vi "Cangrabber.vi"(8 "rt fifo":refnum<k33>) -> ()   [LabVIEW 2014]
uses:
  TeleopCmd.ctl
  CmdFlag.ctl
  <vilib>/Rock Robotics/Network Tables/SD Read Number.vi
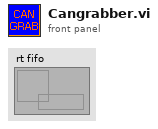
[diagram p1: front panel]
types:
  T1 = typedef "WPI_MotorControlDeviceRef.ctl" = cluster{"DeviceStatus":errorcluster, "Type":T2, "PWM":cluster{"Controller":T3, "PWM Channel":T4, "DeadBand":T5}, "CAN":cluster{"Device Number":u8, "Control Mode":T6, "Semaphore":T7, "Max Vout":dbl, "TalonSRX Control Mode":T8}, "Invert":bool, "TransformRef":T9, "InvTransformRef":T9}
  T2 = typedef "WPI_MotorControlType.ctl" = enum16{"PWM", "CAN", "CANTalonSRX"}
  T3 = typedef "FPGA_TypedefDigitalModule.ctl" = enum16{"Controller 1"}
  T4 = typedef "FPGA_DIOPWMChannel.ctl" = enum8{"PWM 0", "PWM 1", "PWM 2", "PWM 3", "PWM 4", "PWM 5", "PWM 6", "PWM 7", "PWM 8", "PWM 9", "PWM MXP 0", "PWM MXP 1", "PWM MXP 2", "PWM MXP 3", "PWM MXP 4", "PWM MXP 5", "PWM MXP 6", "PWM MXP 7", "PWM MXP 8", "PWM MXP 9", "Invalid"}
  T5 = typedef "WPI_PWMDeadband.ctl" = cluster{"Name":string, "maxPositivePwm":i32, "minPositivePwm":i32, "centerPwm":i32, "maxNegativePwm":i32, "minNegativePwm":i32, "angularRange":u16}
  T6 = typedef "WPI_CANJaguar_ControlMode.ctl" = enum8{"Percent VBus", "Current", "Speed", "Position", "Voltage"}
  T7 = typedef "Semaphore RefNum" = refnum<k1>
  T8 = typedef "WPI_CANTalonSRX_APIControlMode.ctl" = enum8{"Percent VBus", "Speed", "Position", "Slave", "Unchanged / Invalid"}
  T9 = typedef "WPI_PWMTransform_ConPane.ctl" = refnum<vi>
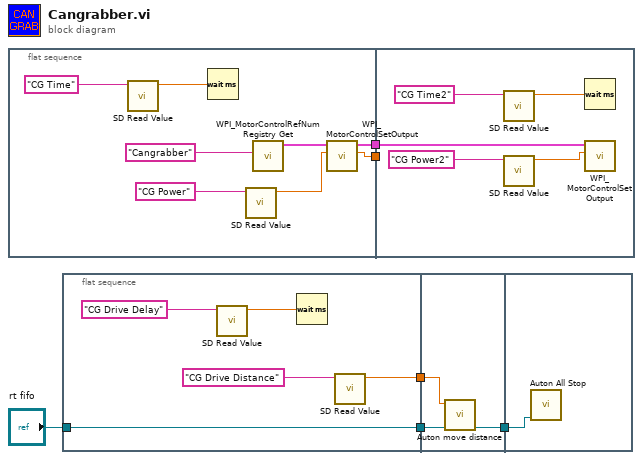
[diagram p0: block diagram]
diagram:
  n1 = flat-sequence {
    tunnel: [w12] -> w6
    tunnel: [w11] -> w5
    tunnel: w6 -> [_]
    tunnel: w5 -> [w19]
    frame #0 {
      n2 = call-poly <vilib>:"SD Read Value.vi"("Name"="CG Time") -> ("Numeric"=w10:dbl)  [unwired: 8 in, 2 out]
      n3 = Wait (ms)(milliseconds to wait=w10) -> ()  [unwired: 1 out]
      n4 = call-poly <vilib>:"SD Read Value.vi"("Name"="CG Power") -> ("Numeric"=w8:dbl)  [unwired: 8 in, 2 out]
      n5 = call <vilib>:"WPI_MotorControlRefNum Registry Get.vi"("refnum name"="Cangrabber") -> ("MotorControlDevRef"=w13:T1)  [unwired: 9 in, 1 out]
      n6 = call <vilib>:"WPI_MotorControlSetOutput.vi"("Output"=w8, "MotorControlDevRef"=w13) -> ("Motor Output"=w12:dbl, "MotorControlDevRef"=w11:T1)  [unwired: 7 in, 1 out]
    }
    frame #1 {
      n7 = call-poly <vilib>:"SD Read Value.vi"("Name"="CG Time2") -> ("Numeric"=w18:dbl)  [unwired: 8 in, 2 out]
      n8 = call-poly <vilib>:"SD Read Value.vi"("Name"="CG Power2") -> ("Numeric"=w17:dbl)  [unwired: 8 in, 2 out]
      n9 = Wait (ms)(milliseconds to wait=w18) -> ()  [unwired: 1 out]
      n10 = call <vilib>:"WPI_MotorControlSetOutput.vi"("Output"=w17, "MotorControlDevRef"=w19) -> ()  [unwired: 7 in, 3 out]
    }
  }
  n11 = flat-sequence {
    tunnel: "rt fifo" -> [w22]
    tunnel: [w22] -> w4
    tunnel: [w20] -> w2
    tunnel: w4 -> [w27]
    tunnel: w2 -> [w26]
    tunnel: [w25] -> w1
    tunnel: w1 -> [w28]
    frame #0 {
      n12 = call-poly <vilib>:"SD Read Value.vi"("Name"="CG Drive Delay") -> ("Numeric"=w24:dbl)  [unwired: 8 in, 2 out]
      n13 = Wait (ms)(milliseconds to wait=w24) -> ()  [unwired: 1 out]
      n14 = call-poly <vilib>:"SD Read Value.vi"("Name"="CG Drive Distance") -> ("Numeric"=w20:dbl)  [unwired: 8 in, 2 out]
    }
    frame #1 {
      n15 = call "Auton move distance.vi"("Distance"=w26, "Refnum in"=w27) -> ("rt fifo out"=w25:refnum<k33>)  [unwired: 7 in, 1 out]
    }
    frame #2 {
      n16 = call "Auton All Stop.vi"("Refnum in"=w28) -> ()  [unwired: 10 in, 1 out]
    }
  }
